vi "PassTactic_Init.vi"(0 "object in":refnum<class "PassTactic.lvclass">, 5 "error in (no error)":errorcluster) -> (14 "object out":refnum<class "PassTactic.lvclass">, 19 "error out":errorcluster)   [LabVIEW 2023, in "PassTactic.lvclass"]
uses:
  PassTactic.lvclass
  C:/Users/ebert/Documents/codes/SSL/repo/SSL_AI/KickTactic_class/KickTactic.lvclass
  C:/Users/ebert/Documents/codes/SSL/repo/SSL_AI/NewSTP/NewTactics/Tactic_v2_class/Tactic_v2.lvclass
  KickTactic_class/KickTactic_states_class/KickTactic_states.ctl
  PassSkill_class/PassSkill.lvclass
  C:/Users/ebert/Documents/codes/SSL/repo/SSL_AI/NewSTP/NewSkills/Skill_v2_class/Skill_v2.lvclass
  NewSTP/NewSkills/Skill_v2_class/Skill_v2.lvclass
  KickTactic_class/KickTactic.lvclass
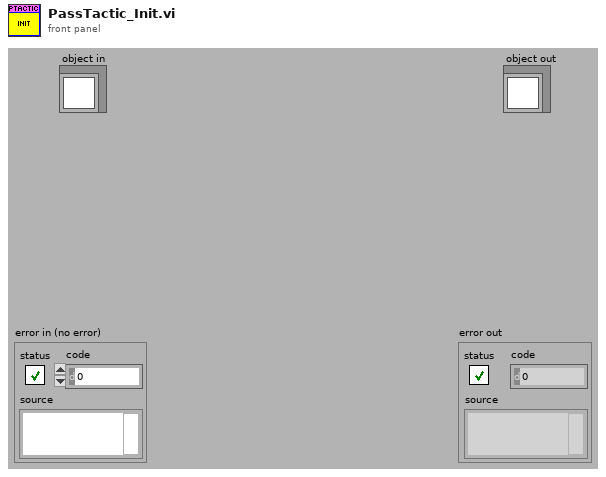
[diagram p1: front panel]
types:
  T1 = typedef "KickTactic.lvclass/KickTactic_states.ctl" = enum16{"GoToTangentPoint", "Circulate", "Align", "Kick"}
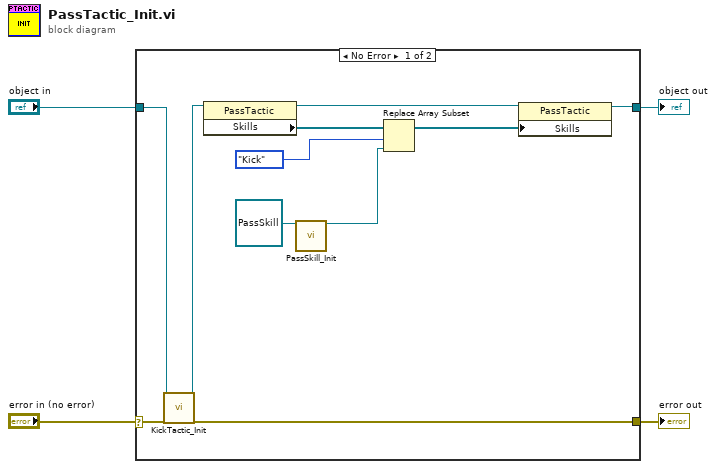
[diagram p0: block diagram]
diagram:
  n1 = case shown="No Error" "error in (no error)" {
    selector: "error in (no error)" -> [w15 w16]
    tunnel: [w12 w17] -> w4
    tunnel: "object in" -> [w13 w17]
    tunnel: [w14 w16] -> w1
    frame No Error {
      n2 = call "KickTactic_Init.vi"("object in"=w13, "error in (no error)"=w15) -> ("object out"=w11:refnum<class "PassTactic.lvclass">, "error out"=w14:errorcluster)  [unwired: 16 in]
      n3 = property class="PassTactic"(reference=w11) -> (reference out=w10:refnum<class "PassTactic.lvclass">, "Skills"=w9:refnum<class "Skill_v2.lvclass">[])  [unwired: 1 in, 1 out]
      n4 = call "PassSkill_Init.vi"("object in"=refnum<class "PassSkill.lvclass"> refnum ("PassSkill")) -> ("object out"=w6:refnum<class "PassSkill.lvclass">)  [unwired: 17 in, 1 out]
      n5 = Replace Array Subset(array=w9, new element=w6, index=KickTactic_states."Kick" ("Enum")) -> (w5:refnum<class "Skill_v2.lvclass">[])
      n6 = property class="PassTactic"(reference=w10, "Skills"=w5) -> (reference out=w12:refnum<class "PassTactic.lvclass">)  [unwired: 1 in, 1 out]
    }
    frame Error {
    }
  }
  "object out" <- w4
  "error out" <- w1
